vi "Read Helper.vi"(11 "Panel in":refnum<class "Panel.lvclass">) -> (2 "Helper":refnum<class "Panel Helper.lvclass">)   [LabVIEW 2019, in "Panel.lvlib" / "Panel.lvclass"]
doc: "Reads the panel helper for this panel object.\n----\nCopyright: MGI 2017\nAuthor: Derek Trepanier"
uses:
  Panel.lvclass
  Panel Helper/Panel Helper.lvclass
  Panel.lvclass/Panel.ctl
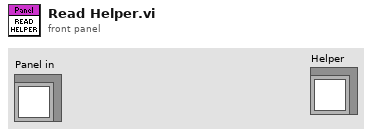
[diagram p1: front panel]
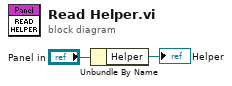
[diagram p0: block diagram]
diagram:
  n1 = Unbundle By Name("Panel in") -> ("Helper"=→"Helper":refnum<class "Panel Helper.lvclass">)
